vi "Show Dialog.vi"(8 "error in (no error)":errorcluster, 11 "Dialog in":refnum<class "Dialog.lvclass">) -> (0 "error out":errorcluster, 3 "Dialog out":refnum<class "Dialog.lvclass">)   [LabVIEW 2020, in "Dialog Classes.lvlib" / "Dialog.lvclass"]
uses:
  Dialog.lvclass
  Dialog.lvclass/Dialog.ctl
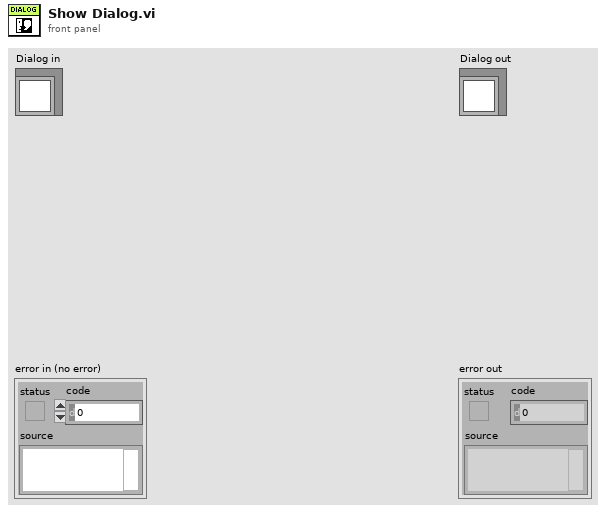
[diagram p1: front panel]
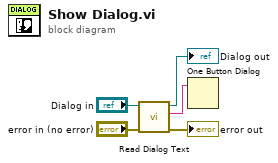
[diagram p0: block diagram]
diagram:
  n1 = call "Read Dialog Text.vi"("error in (no error)"="error in (no error)", "Dialog in"="Dialog in") -> ("error out"=→"error out":errorcluster, "Dialog Text"=w1:string, "Dialog out"=→"Dialog out":refnum<class "Dialog.lvclass">)  [unwired: 7 in]
  n2 = One Button Dialog(message=w1) -> ()  [unwired: 1 in, 1 out]
